vi "ListInstruments.vi"(8 "error in (no error)":errorcluster, 11 "PalmSens in":refnum<class "PalmSens.lvclass">) -> (0 "error out":errorcluster, 2 "Array":string[](array[string]), 3 "PalmSens out":refnum<class "PalmSens.lvclass">)   [LabVIEW 2025, in "PalmSens.lvclass"]
uses:
  PalmSens.lvclass
  PalmSens.lvclass/PalmSens.ctl
  E:/PSCode/PalmSens_SDK/labview/PalmSens/Libraries/PalmSens.Core.Simplified.LabVIEW.dll
  Libraries/PalmSens.Core.Simplified.LabVIEW.dll
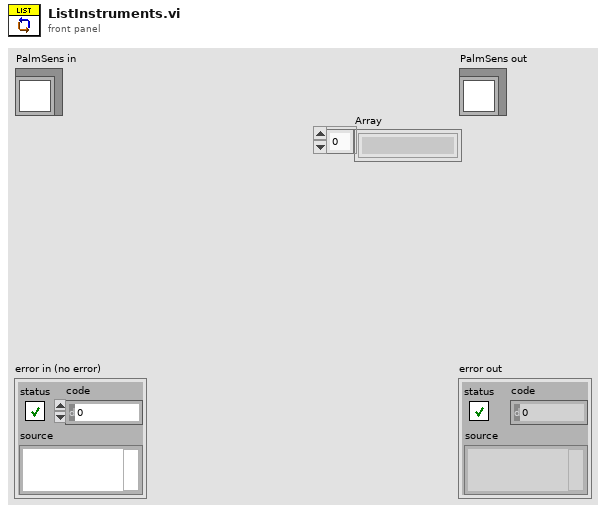
[diagram p1: front panel]
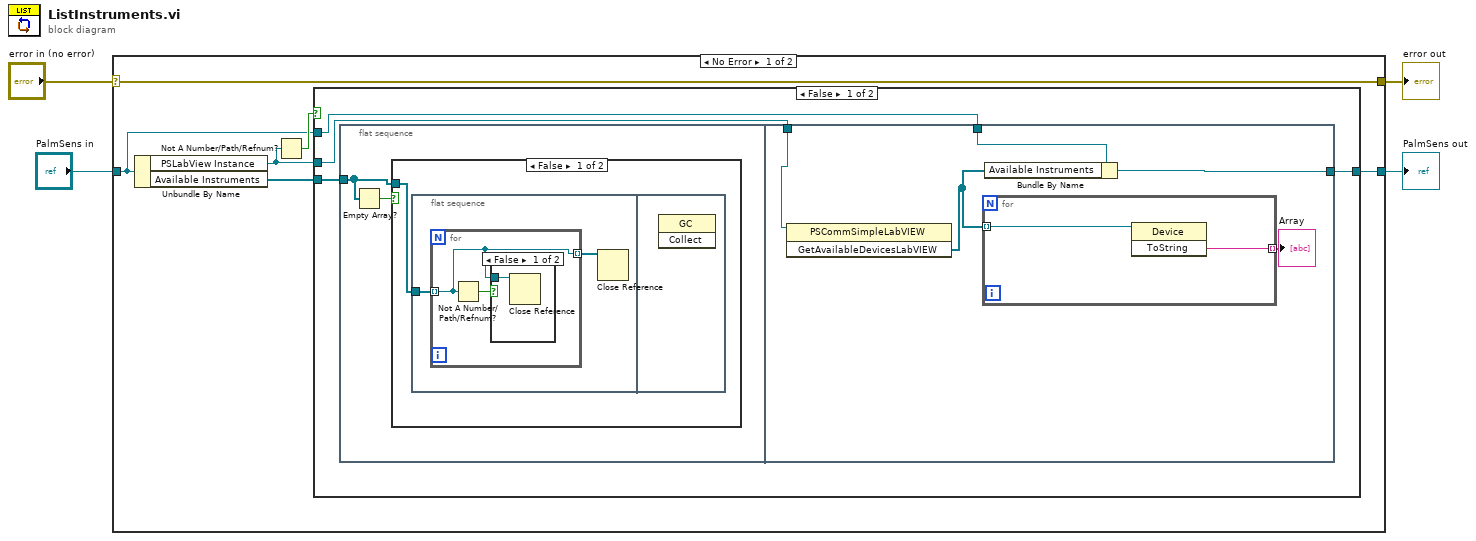
[diagram p0: block diagram]
diagram:
  n1 = case shown="No Error" "error in (no error)" {
    selector: "error in (no error)" -> [w10 w32]
    tunnel: [w10 w32] -> w3
    tunnel: [w5 w31] -> w2
    tunnel: "PalmSens in" -> [w6 w31]
    frame No Error {
      n2 = Unbundle By Name(w6) -> ("PSLabView Instance"=w7:refnum<k24>, "Available Instruments"=w9:refnum<k24>[])
      n3 = Not A Number/Path/Refnum?(number/path/refnum=w7) -> (NaN/Path/Refnum?=w8:bool)
      n4 = case shown="False" w8 {
        tunnel: w9 -> [w14 _]
        tunnel: w7 -> [w13 _]
        tunnel: [w12 w30] -> w5
        tunnel: w6 -> [w11 w30]
        frame False {
          n5 = flat-sequence {
            tunnel: w14 -> [w16]
            tunnel: w13 -> [w24]
            tunnel: [w27] -> w12
            tunnel: w11 -> [w26]
            frame #0 {
              n6 = Empty Array?(array=w16) -> (empty?=w15:bool)
              n7 = case shown="False" w15 {
                tunnel: w16 -> [w17 _]
                frame False {
                  n8 = flat-sequence {
                    tunnel: w17 -> [w18]
                    frame #0 {
                      n9 = for {
                        tunnel: w18 -> [w21] mode=indexing
                        tunnel: [w21] -> w19 mode=indexing
                        n10 = Not A Number/Path/Refnum?(number/path/refnum=w21) -> (NaN/Path/Refnum?=w20:bool)
                        n11 = case shown="False" w20 {
                          tunnel: w21 -> [w22 _]
                          frame False {
                            n12 = Close Reference(reference=w22) -> ()  [unwired: 1 in, 1 out]
                          }
                          frame True {
                          }
                        }
                      }
                      n13 = Close Reference(reference=w19) -> ()  [unwired: 1 in, 1 out]
                    }
                    frame #1 {
                      n14 = invoke class="GC" method="Collect"() -> ()  [unwired: 3 in, 3 out]
                    }
                  }
                }
                frame True {
                }
              }
            }
            frame #1 {
              n15 = invoke class="PSCommSimpleLabVIEW" method="GetAvailableDevicesLabVIEW"(reference=w24) -> ("GetAvailableDevicesLabVIEW"=w23:refnum<k24>[])  [unwired: 2 in, 2 out]
              n16 = for {
                tunnel: w23 -> [w29] mode=indexing
                tunnel: [w28] -> w25 mode=indexing
                n17 = invoke class="Device" method="ToString"(reference=w29) -> ("ToString"=w28:string)  [unwired: 2 in, 2 out]
              }
              "Array" <- w25
              n18 = Bundle By Name(cluster=w26, "Available Instruments"=w23) -> (w27:refnum<class "PalmSens.lvclass">)
            }
          }
        }
        frame True {
        }
      }
    }
    frame Error {
    }
  }
  "error out" <- w3
  "PalmSens out" <- w2
